vi "Get Splitter Position.vi"(8 "error in (no error)":errorcluster, 11 "Interaction Splitter in":refnum<class "Interaction Splitter.lvclass">) -> (0 "error out":errorcluster, 2 "Splitter Position":i32, 3 "Interaction Splitter out":refnum<class "Interaction Splitter.lvclass">)   [LabVIEW 2013, in "Interaction Splitter.lvclass"]
doc: "Copyright 2018, Wiebe Walstra, wiebe@carya.nl."
uses:
  Interaction Splitter.lvclass
  Interaction Splitter.lvclass/Interaction Splitter.ctl
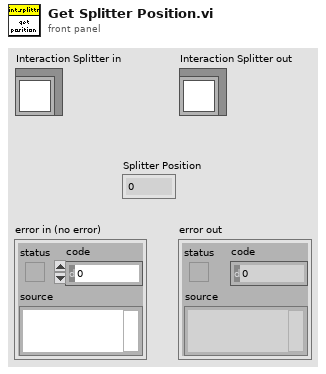
[diagram p1: front panel]
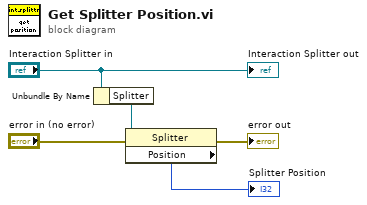
[diagram p0: block diagram]
diagram:
  n1 = Unbundle By Name("Interaction Splitter in") -> ("Splitter"=w2:refnum<vi>)
  n2 = property class="Splitter"(reference=w2, error in="error in (no error)") -> (error out=→"error out":errorcluster, "Position"=→"Splitter Position":i32)  [unwired: 1 out]
  "Interaction Splitter out" <- "Interaction Splitter in"
